vi "总磷总氮测量数据储存.vi"   [LabVIEW 2016, in "斯坦道氨氮.lvlib"]
types:
  T1 = cluster{"时间标识":timestamp, "测量模式":enum16{"维护数据", "水样测试", "标样核查", "零点核查", "跨度核查", "空白测试", "平行样测试", "加标回收", "空白校准", "标样校准", "初始化（清洗）"}, "数据标记表":string, "监测值":sgl, "单位":u16, "数据标识":string, "因子编码":u32, "标样参考值":sgl, "F0":sgl, "F1":sgl, "F2":sgl, "F3":sgl, "F4":sgl, "F5":sgl, "F6":sgl, "F7":sgl, "X":sgl, "温度":sgl, "湿度":sgl, "量程标识":string, "SN":string, "跨度值":sgl}
  T2 = enum16{"维护数据", "水样测试", "标样核查", "零点核查", "跨度核查", "空白测试", "平行样测试", "加标回收", "空白校准", "标样校准", "初始化（清洗）"}
  T3 = cluster{"系统时间":timestamp, "工作状态":enum16{"空闲", "水样测试", "标样核查", "零点核查", "跨度核查", "空白测试", "平行样测试", "加标回收", "空白校准", "标样校准", "初始化（清洗）"}, "测量模式":enum16{"待机", "连续模式", "周期模式", "定点模式", "受控模式", "手动模式"}, "告警代码":u16, "故障代码":u16, "日志代码":u16, "软件版本":u16, "F0":sgl, "F1":sgl, "F2":sgl, "F3":sgl, "T":sgl, "H":sgl, "id":u16, "flowid":u16, "量程":u16, "总磷控温温度1":sgl, "营养盐控温温度2":sgl, "ADC":sgl}
  T4 = cluster{"运行模式":enum16{"维护模式", "常规模式", "应急模式", "质控模式"}, "质控频次":enum16{"关闭", "每天", "星期一", "星期二", "星期三", "星期四", "星期五", "星期六", "星期日"}, "空白核查时间":u16, "跨度核查时间":u16, "24H周期设置":bool[]}
  T5 = enum16{"空闲", "水样测试", "标样核查", "零点核查", "跨度核查", "空白测试", "平行样测试", "加标回收", "空白校准", "标样校准", "初始化（清洗）"}
  T6 = cluster{"因子编码":u32, "单位":u16, "标样参考值":sgl, "水样数据时间":timestamp, "水样实测值":sgl, "水样数据标识":string, "标样数据时间":timestamp, "标样实测值":sgl, "标样数据标识":string, "空白数据时间":timestamp, "空白实测值":sgl, "空白数据标识":string, "零点核查数据时间":timestamp, "零点核查实测值":sgl, "零点核查数据标识":string, "跨度核查数据时间":timestamp, "跨度核查实测值":sgl, "跨度核查数据标识":string, "加标回收数据时间":timestamp, "加标回收实测值":sgl, "加标回收数据标识":string, "平行样数据时间":timestamp, "平行样实测值":sgl, "平行样数据标识":string, "F0":sgl, "F1":sgl, "F2":sgl, "F3":sgl, "F4":sgl, "F5":sgl, "F6":sgl, "F7":sgl, "温度":sgl, "湿度":sgl, "X值":sgl, "fidrange":u16}
  T7 = cluster{"总磷跨度值":dbl, "总磷零点标准液浓度":dbl, "总磷跨度标准液浓度":dbl, "总磷标准液标准浓度":dbl, "总氮跨度值":dbl, "总氮零点标准液浓度":dbl, "总氮跨度标准液浓度":dbl, "总氮标准液标准浓度":dbl, "COD跨度值":dbl, "COD零点标准液浓度":dbl, "COD跨度标准液浓度":dbl, "COD标准液标准浓度":dbl, "氨氮跨度值":dbl, "氨氮零点标准液浓度":dbl, "氨氮跨度标准液浓度":dbl, "氨氮标准液标准浓度":dbl}
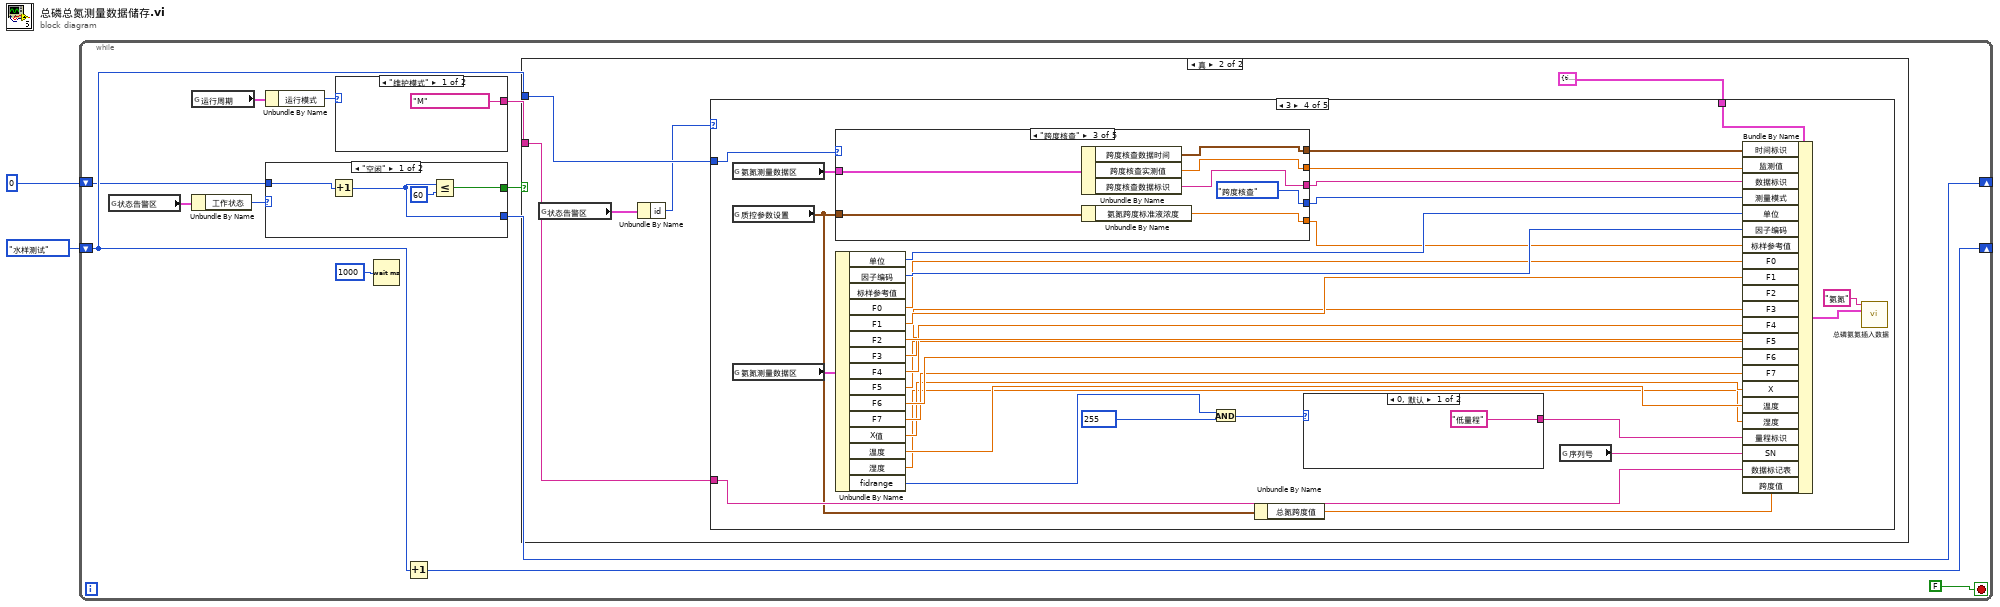
[diagram p0: block diagram]
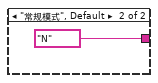
[diagram p3: hidden frame]
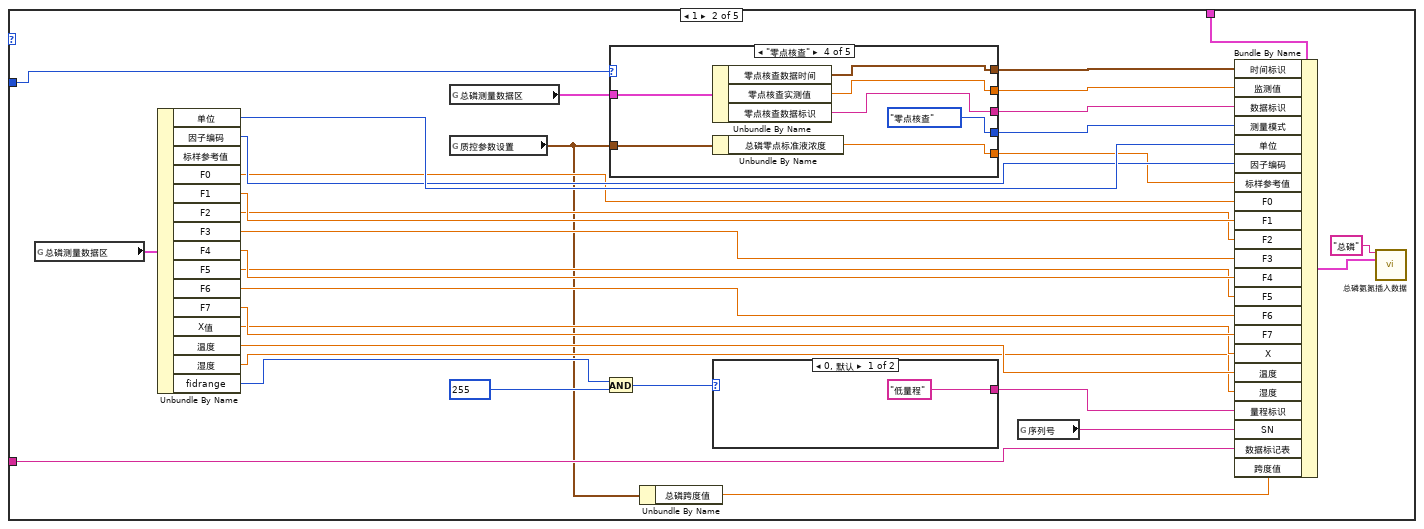
[diagram p6: hidden frame]
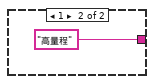
[diagram p7: hidden frame]
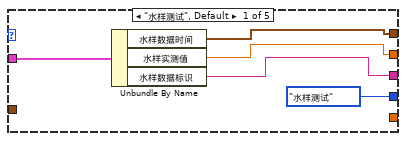
[diagram p8: hidden frame]
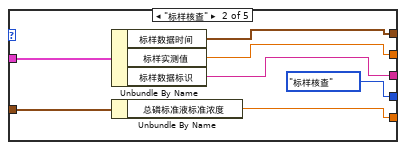
[diagram p9: hidden frame]
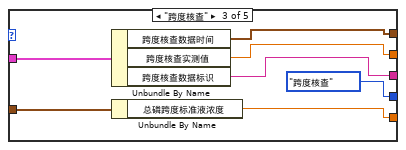
[diagram p10: hidden frame]
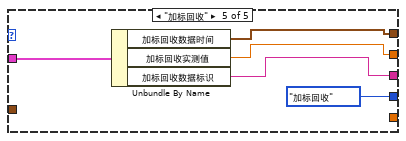
[diagram p11: hidden frame]
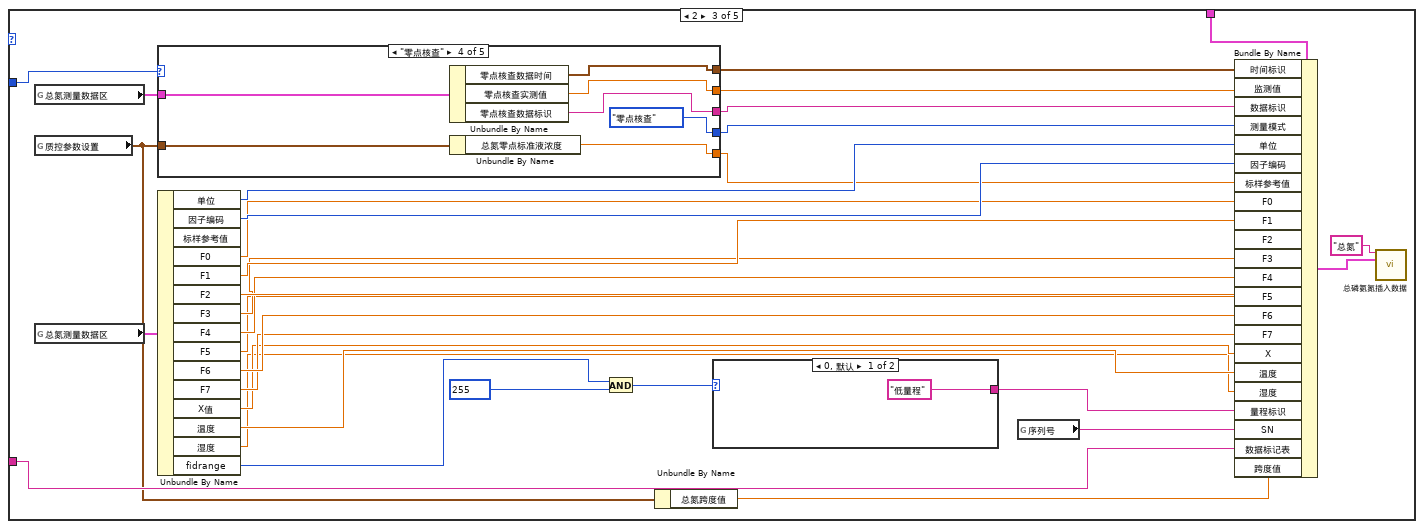
[diagram p12: hidden frame]
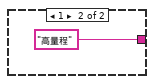
[diagram p13: hidden frame]
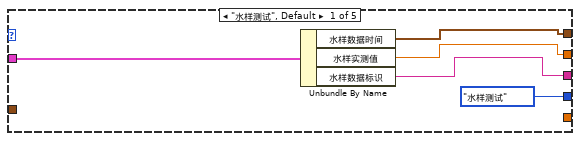
[diagram p14: hidden frame]
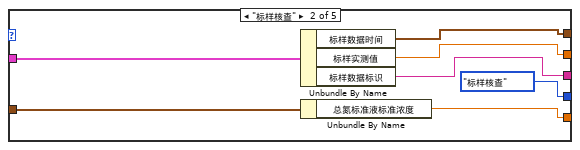
[diagram p15: hidden frame]
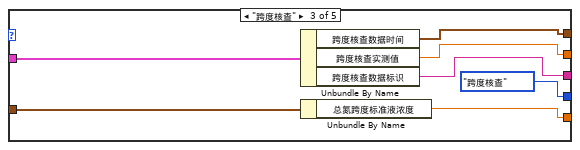
[diagram p16: hidden frame]
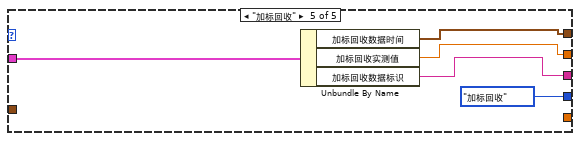
[diagram p17: hidden frame]
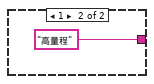
[diagram p18: hidden frame]
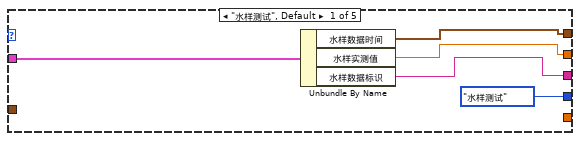
[diagram p19: hidden frame]
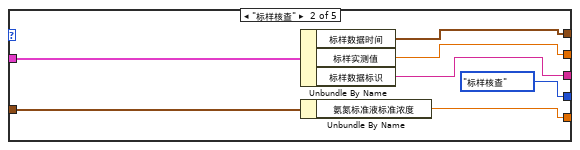
[diagram p20: hidden frame]
diagram:
  n1 = while {
    shift-right: [w12] -> _
    shift-left: enum16{"水样测试", "标样核查", "跨度核查", "零点核查", "加标回收"}."水样测试" ("测量模式") -> [w11]
    shift-right: [w5] -> _
    shift-left: u32 0 ("等待时间（毫秒）") -> [w6]
    stop <- FALSE stop-if-true
    n2 = global read "VAR总磷总氮全局变量.vi" "状态告警区"() -> (w8:T3)
    n3 = global read "总磷总氮断电保存全局变量.vi" "运行周期"() -> (w10:T4)
    n4 = Unbundle By Name(w8) -> ("工作状态"=w7:T5)
    n5 = Unbundle By Name(w10) -> ("运行模式"=w9:enum16{"维护模式", "常规模式", "应急模式", "质控模式"})
    n6 = case shown="\"空闲\"" w7 {
      tunnel: w6 -> [w18 _]
      tunnel: [w17 _] -> w5
      tunnel: [w15 _] -> w4
      frame "空闲" {
        n7 = Increment(x=w18) -> (x+1=w17:u32)
        n8 = Less Or Equal?(x=w17, y=u32 60) -> (x <= y?=w15:bool)
      }
      frame "水样测试", Default {
      }
    }
    n9 = case shown="\"维护模式\"" w9 {
      tunnel: ["M" ("数据标记表") "N" ("数据标记表")] -> w13
      frame "维护模式" {
      }
      frame "常规模式", Default {
      }
    }
    n10 = Wait (ms)(milliseconds to wait=u32 1000 ("等待时间（毫秒）")) -> ()  [unwired: 1 out]
    n11 = Increment(x=w11) -> (x+1=w12:enum16{"水样测试", "标样核查", "跨度核查", "零点核查", "加标回收"})
    n12 = case shown="真" w4 {
      tunnel: w13 -> [_ w25]
      tunnel: w11 -> [_ w24]
      frame False {
      }
      frame True {
        n13 = global read "VAR总磷总氮全局变量.vi" "状态告警区"() -> (w23:T3)
        n14 = Unbundle By Name(w23) -> ("id"=w22:u16)
        n15 = case shown="3" w22 {
          tunnel: w25 -> [_ w30 w95 w160 w226]
          tunnel: w24 -> [_ w39 w108 w173 w238]
          tunnel: T1 {"时间标识"=timestamp(0 s since 1904-01-01), "测量模式"=enum."水样测试", "数据标记表"="N", "监测值"=0.0, "单位"=0, "数据标识"="", "因子编码"=0, "标样参考值"=0.0, "F0"=0.0, "F1"=0.0, "F2"=0.0, "F3"=0.0, "F4"=0.0, "F5"=0.0, "F6"=0.0, "F7"=0.0, "X"=0.0, "温度"=0.0, "湿度"=0.0, "量程标识"="", "SN"="", "跨度值"=0.0} ("data") -> [_ w28 w93 w158 w224]
          frame Default {
          }
          frame 1 {
            n16 = global read "VAR总磷总氮全局变量.vi" "总磷测量数据区"() -> (w43:T6)
            n17 = Unbundle By Name(w43) -> ("单位"=w56:u16, "因子编码"=w55:u32, "F0"=w54:sgl, "F1"=w53:sgl, "F2"=w52:sgl, "F3"=w51:sgl, "F4"=w50:sgl, "F5"=w49:sgl, "F6"=w48:sgl, "F7"=w47:sgl, "X值"=w46:sgl, "温度"=w45:sgl, "湿度"=w44:sgl, "fidrange"=w37:u16)  [unwired: 1 out]
            n18 = global read "VAR总磷总氮全局变量.vi" "总磷测量数据区"() -> (w57:T6)
            n19 = global read "总磷总氮断电保存全局变量.vi" "质控参数设置"() -> (w27:T7)
            n20 = And(x=w37, y=u16 255) -> (x .and. y?=w35:u16)
            n21 = case shown="\"零点核查\"" w39 {
              tunnel: w57 -> [w64 w71 w78 w85 w90]
              tunnel: [w63 w70 w77 w84 w89] -> w40
              tunnel: [w62 w69 w76 w83 w88] -> w41
              tunnel: [w61 w68 w75 w82 w87] -> w42
              tunnel: [T2."水样测试" ("测量模式") T2."标样核查" ("测量模式") T2."跨度核查" ("测量模式") T2."零点核查" ("测量模式") T2."加标回收" ("测量模式")] -> w29
              tunnel: w27 -> [_ w66 w73 w80 _]
              tunnel: [_ w65 w72 w79 _] -> w38
              frame "水样测试", Default {
                n22 = Unbundle By Name(w64) -> ("水样数据时间"=w63:timestamp, "水样实测值"=w62:sgl, "水样数据标识"=w61:string)
              }
              frame "标样核查" {
                n23 = Unbundle By Name(w71) -> ("标样数据时间"=w70:timestamp, "标样实测值"=w69:sgl, "标样数据标识"=w68:string)
                n24 = Unbundle By Name(w66) -> ("总磷标准液标准浓度"=w65:dbl)
              }
              frame "跨度核查" {
                n25 = Unbundle By Name(w78) -> ("跨度核查数据时间"=w77:timestamp, "跨度核查实测值"=w76:sgl, "跨度核查数据标识"=w75:string)
                n26 = Unbundle By Name(w73) -> ("总磷跨度标准液浓度"=w72:dbl)
              }
              frame "零点核查" {
                n27 = Unbundle By Name(w85) -> ("零点核查数据时间"=w84:timestamp, "零点核查实测值"=w83:sgl, "零点核查数据标识"=w82:string)
                n28 = Unbundle By Name(w80) -> ("总磷零点标准液浓度"=w79:dbl)
              }
              frame "加标回收" {
                n29 = Unbundle By Name(w90) -> ("加标回收数据时间"=w89:timestamp, "加标回收实测值"=w88:sgl, "加标回收数据标识"=w87:string)
              }
            }
            n30 = Unbundle By Name(w27) -> ("总磷跨度值"=w26:dbl)
            n31 = case shown="0, 默认" w35 {
              tunnel: ["低量程" ("格式字符串") "高量程" ("格式字符串")] -> w34
              frame 0, Default {
              }
              frame 1 {
              }
            }
            n32 = global read "VAR总磷总氮全局变量.vi" "序列号"() -> (w31:string)
            n33 = Bundle By Name(cluster=w28, "时间标识"=w40, "监测值"=w41, "数据标识"=w42, "测量模式"=w29, "单位"=w56, "因子编码"=w55, "标样参考值"=w38, "F0"=w54, "F1"=w53, "F2"=w52, "F3"=w51, "F4"=w50, "F5"=w49, "F6"=w48, "F7"=w47, "X"=w46, "温度"=w45, "湿度"=w44, "量程标识"=w34, "SN"=w31, "数据标记表"=w30, "跨度值"=w26) -> (w32:T1)
            n34 = call "总磷氨氮插入数据.vi"("table"="总磷", "data"=w32) -> ()  [unwired: 13 in, 1 out]
          }
          frame 2 {
            n35 = global read "VAR总磷总氮全局变量.vi" "总氮测量数据区"() -> (w107:T6)
            n36 = global read "总磷总氮断电保存全局变量.vi" "质控参数设置"() -> (w92:T7)
            n37 = global read "VAR总磷总氮全局变量.vi" "总氮测量数据区"() -> (w122:T6)
            n38 = case shown="\"零点核查\"" w108 {
              tunnel: w107 -> [w129 w136 w143 w150 w155]
              tunnel: [w128 w135 w142 w149 w154] -> w106
              tunnel: [w127 w134 w141 w148 w153] -> w105
              tunnel: [w126 w133 w140 w147 w152] -> w104
              tunnel: [T2."水样测试" ("测量模式") T2."标样核查" ("测量模式") T2."跨度核查" ("测量模式") T2."零点核查" ("测量模式") T2."加标回收" ("测量模式")] -> w94
              tunnel: w92 -> [_ w131 w138 w145 _]
              tunnel: [_ w130 w137 w144 _] -> w103
              frame "水样测试", Default {
                n39 = Unbundle By Name(w129) -> ("水样数据时间"=w128:timestamp, "水样实测值"=w127:sgl, "水样数据标识"=w126:string)
              }
              frame "标样核查" {
                n40 = Unbundle By Name(w136) -> ("标样数据时间"=w135:timestamp, "标样实测值"=w134:sgl, "标样数据标识"=w133:string)
                n41 = Unbundle By Name(w131) -> ("总氮标准液标准浓度"=w130:dbl)
              }
              frame "跨度核查" {
                n42 = Unbundle By Name(w143) -> ("跨度核查数据时间"=w142:timestamp, "跨度核查实测值"=w141:sgl, "跨度核查数据标识"=w140:string)
                n43 = Unbundle By Name(w138) -> ("总氮跨度标准液浓度"=w137:dbl)
              }
              frame "零点核查" {
                n44 = Unbundle By Name(w150) -> ("零点核查数据时间"=w149:timestamp, "零点核查实测值"=w148:sgl, "零点核查数据标识"=w147:string)
                n45 = Unbundle By Name(w145) -> ("总氮零点标准液浓度"=w144:dbl)
              }
              frame "加标回收" {
                n46 = Unbundle By Name(w155) -> ("加标回收数据时间"=w154:timestamp, "加标回收实测值"=w153:sgl, "加标回收数据标识"=w152:string)
              }
            }
            n47 = Unbundle By Name(w122) -> ("单位"=w121:u16, "因子编码"=w120:u32, "F0"=w119:sgl, "F1"=w118:sgl, "F2"=w117:sgl, "F3"=w116:sgl, "F4"=w115:sgl, "F5"=w114:sgl, "F6"=w113:sgl, "F7"=w112:sgl, "X值"=w111:sgl, "温度"=w110:sgl, "湿度"=w109:sgl, "fidrange"=w100:u16)  [unwired: 1 out]
            n48 = And(x=w100, y=u16 255) -> (x .and. y?=w101:u16)
            n49 = Unbundle By Name(w92) -> ("总氮跨度值"=w91:dbl)
            n50 = case shown="0, 默认" w101 {
              tunnel: ["低量程" ("格式字符串") "高量程" ("格式字符串")] -> w99
              frame 0, Default {
              }
              frame 1 {
              }
            }
            n51 = global read "VAR总磷总氮全局变量.vi" "序列号"() -> (w96:string)
            n52 = Bundle By Name(cluster=w93, "时间标识"=w106, "监测值"=w105, "数据标识"=w104, "测量模式"=w94, "单位"=w121, "因子编码"=w120, "标样参考值"=w103, "F0"=w119, "F1"=w118, "F2"=w117, "F3"=w116, "F4"=w115, "F5"=w114, "F6"=w113, "F7"=w112, "X"=w111, "温度"=w110, "湿度"=w109, "量程标识"=w99, "SN"=w96, "数据标记表"=w95, "跨度值"=w91) -> (w98:T1)
            n53 = call "总磷氨氮插入数据.vi"("table"="总氮", "data"=w98) -> ()  [unwired: 13 in, 1 out]
          }
          frame 3 {
            n54 = global read "VAR总磷总氮全局变量.vi" "氨氮测量数据区"() -> (w172:T6)
            n55 = global read "总磷总氮断电保存全局变量.vi" "质控参数设置"() -> (w157:T7)
            n56 = global read "VAR总磷总氮全局变量.vi" "氨氮测量数据区"() -> (w187:T6)
            n57 = case shown="\"跨度核查\"" w173 {
              tunnel: w172 -> [w194 w201 w208 w215 w220]
              tunnel: [w193 w200 w207 w214 w219] -> w171
              tunnel: [w192 w199 w206 w213 w218] -> w170
              tunnel: [w191 w198 w205 w212 w217] -> w169
              tunnel: [T2."水样测试" ("测量模式") T2."标样核查" ("测量模式") T2."跨度核查" ("测量模式") T2."零点核查" ("测量模式") T2."加标回收" ("测量模式")] -> w159
              tunnel: w157 -> [_ w196 w203 w210 _]
              tunnel: [_ w195 w202 w209 _] -> w168
              frame "水样测试", Default {
                n58 = Unbundle By Name(w194) -> ("水样数据时间"=w193:timestamp, "水样实测值"=w192:sgl, "水样数据标识"=w191:string)
              }
              frame "标样核查" {
                n59 = Unbundle By Name(w201) -> ("标样数据时间"=w200:timestamp, "标样实测值"=w199:sgl, "标样数据标识"=w198:string)
                n60 = Unbundle By Name(w196) -> ("氨氮标准液标准浓度"=w195:dbl)
              }
              frame "跨度核查" {
                n61 = Unbundle By Name(w208) -> ("跨度核查数据时间"=w207:timestamp, "跨度核查实测值"=w206:sgl, "跨度核查数据标识"=w205:string)
                n62 = Unbundle By Name(w203) -> ("氨氮跨度标准液浓度"=w202:dbl)
              }
              frame "零点核查" {
                n63 = Unbundle By Name(w215) -> ("零点核查数据时间"=w214:timestamp, "零点核查实测值"=w213:sgl, "零点核查数据标识"=w212:string)
                n64 = Unbundle By Name(w210) -> ("氨氮零点标准液浓度"=w209:dbl)
              }
              frame "加标回收" {
                n65 = Unbundle By Name(w220) -> ("加标回收数据时间"=w219:timestamp, "加标回收实测值"=w218:sgl, "加标回收数据标识"=w217:string)
              }
            }
            n66 = Unbundle By Name(w187) -> ("单位"=w186:u16, "因子编码"=w185:u32, "F0"=w184:sgl, "F1"=w183:sgl, "F2"=w182:sgl, "F3"=w181:sgl, "F4"=w180:sgl, "F5"=w179:sgl, "F6"=w178:sgl, "F7"=w177:sgl, "X值"=w176:sgl, "温度"=w175:sgl, "湿度"=w174:sgl, "fidrange"=w165:u16)  [unwired: 1 out]
            n67 = And(x=w165, y=u16 255) -> (x .and. y?=w166:u16)
            n68 = Unbundle By Name(w157) -> ("总氮跨度值"=w156:dbl)
            n69 = case shown="0, 默认" w166 {
              tunnel: ["低量程" ("格式字符串") "高量程" ("格式字符串")] -> w164
              frame 0, Default {
              }
              frame 1 {
              }
            }
            n70 = global read "VAR总磷总氮全局变量.vi" "序列号"() -> (w161:string)
            n71 = Bundle By Name(cluster=w158, "时间标识"=w171, "监测值"=w170, "数据标识"=w169, "测量模式"=w159, "单位"=w186, "因子编码"=w185, "标样参考值"=w168, "F0"=w184, "F1"=w183, "F2"=w182, "F3"=w181, "F4"=w180, "F5"=w179, "F6"=w178, "F7"=w177, "X"=w176, "温度"=w175, "湿度"=w174, "量程标识"=w164, "SN"=w161, "数据标记表"=w160, "跨度值"=w156) -> (w163:T1)
            n72 = call "总磷氨氮插入数据.vi"("table"="氨氮", "data"=w163) -> ()  [unwired: 13 in, 1 out]
          }
          frame 22 {
            n73 = global read "VAR总磷总氮全局变量.vi" "COD测量数据区"() -> (w237:T6)
            n74 = global read "VAR总磷总氮全局变量.vi" "COD测量数据区"() -> (w252:T6)
            n75 = global read "总磷总氮断电保存全局变量.vi" "质控参数设置"() -> (w222:T7)
            n76 = case shown="\"跨度核查\"" w238 {
              tunnel: w237 -> [w259 w266 w273 w280 w285]
              tunnel: [w258 w265 w272 w279 w284] -> w236
              tunnel: [w257 w264 w271 w278 w283] -> w235
              tunnel: [w256 w263 w270 w277 w282] -> w234
              tunnel: [T2."水样测试" ("测量模式") T2."标样核查" ("测量模式") T2."跨度核查" ("测量模式") T2."零点核查" ("测量模式") T2."加标回收" ("测量模式")] -> w225
              tunnel: w222 -> [_ w261 w268 w275 _]
              tunnel: [_ w260 w267 w274 _] -> w233
              frame "水样测试", Default {
                n77 = Unbundle By Name(w259) -> ("水样数据时间"=w258:timestamp, "水样实测值"=w257:sgl, "水样数据标识"=w256:string)
              }
              frame "标样核查" {
                n78 = Unbundle By Name(w261) -> ("COD标准液标准浓度"=w260:dbl)
                n79 = Unbundle By Name(w266) -> ("标样数据时间"=w265:timestamp, "标样实测值"=w264:sgl, "标样数据标识"=w263:string)
              }
              frame "跨度核查" {
                n80 = Unbundle By Name(w268) -> ("COD跨度标准液浓度"=w267:dbl)
                n81 = Unbundle By Name(w273) -> ("跨度核查数据时间"=w272:timestamp, "跨度核查实测值"=w271:sgl, "跨度核查数据标识"=w270:string)
              }
              frame "零点核查" {
                n82 = Unbundle By Name(w275) -> ("COD零点标准液浓度"=w274:dbl)
                n83 = Unbundle By Name(w280) -> ("零点核查数据时间"=w279:timestamp, "零点核查实测值"=w278:sgl, "零点核查数据标识"=w277:string)
              }
              frame "加标回收" {
                n84 = Unbundle By Name(w285) -> ("加标回收数据时间"=w284:timestamp, "加标回收实测值"=w283:sgl, "加标回收数据标识"=w282:string)
              }
            }
            n85 = Unbundle By Name(w252) -> ("单位"=w251:u16, "因子编码"=w250:u32, "F0"=w249:sgl, "F1"=w248:sgl, "F2"=w247:sgl, "F3"=w246:sgl, "F4"=w245:sgl, "F5"=w244:sgl, "F6"=w243:sgl, "F7"=w242:sgl, "X值"=w241:sgl, "温度"=w240:sgl, "湿度"=w239:sgl, "fidrange"=w230:u16)  [unwired: 1 out]
            n86 = Unbundle By Name(w222) -> ("COD跨度值"=w221:dbl)
            n87 = And(x=w230, y=u16 255) -> (x .and. y?=w231:u16)
            n88 = case shown="0, 默认" w231 {
              tunnel: ["低量程" ("格式字符串") "高量程" ("格式字符串")] -> w229
              frame 0, Default {
              }
              frame 1 {
              }
            }
            n89 = global read "VAR总磷总氮全局变量.vi" "序列号"() -> (w227:string)
            n90 = Bundle By Name(cluster=w224, "时间标识"=w236, "监测值"=w235, "数据标识"=w234, "测量模式"=w225, "单位"=w251, "因子编码"=w250, "标样参考值"=w233, "F0"=w249, "F1"=w248, "F2"=w247, "F3"=w246, "F4"=w245, "F5"=w244, "F6"=w243, "F7"=w242, "X"=w241, "温度"=w240, "湿度"=w239, "量程标识"=w229, "SN"=w227, "数据标记表"=w226, "跨度值"=w221) -> (w223:T1)
            n91 = call "总磷氨氮插入数据.vi"("table"="COD", "data"=w223) -> ()  [unwired: 13 in, 1 out]
          }
        }
      }
    }
  }
